vi "OBJ_LOGIN_scan_barcode.vi"(8 "error_in":errorcluster, 11 "all_config_info":T1={"main_ini_file"={"SQL Driver"="", "SQL Server"="", "SQL Database"="", "SQL UID"="", "User table"="", "Reference table"="", "default language"="", "SCANNER COM port"=0, "SCANNER Baud rate"=0, "SCANNER Data bits"=0, "SCANNER Pairity"=enum."None", "SCANNER Stop bits"=10, "SCANNER Flow control"=0, "SCANNER Termination char"=0, "MD-L COM port"=0, "MD-L Baud rate"=0, "MD-L Data bits"=0, "MD-L Pairity"=enum."None", "MD-L Stop bits"=10, "MD-L Flow control"=0, "MD-L Termination char"=0, "MD-R COM port"=0, "MD-R Baud rate"=0, "MD-R Data bits"=0, "MD-R Pairity"=enum."None", "MD-R Stop bits"=10, "MD-R Flow control"=0, "MD-R Termination char"=0, "logout timeout [ms]"=0}, "SQL Password"="", "queue_refnums"={"MAIN_queue"=refnum, "SCANNER_queue"=refnum, "SCANNER_login"=refnum, "MD_L_queue"=refnum, "MD_L_data"=refnum, "MD_R_queue"=refnum, "MD_R_data"=refnum, "OBJ_GUI_TIMER_queue"=refnum}} {"main_ini_file"."MD-R Flow control" items=["None"=0, "XON/XOFF"=1, "RTS/CTS"=2, "DTR/DSR"=4]; "main_ini_file"."MD-R Stop bits" items=["1.0"=10, "1.5"=15, "2.0"=20]; "main_ini_file"."MD-L Flow control" items=["None"=0, "XON/XOFF"=1, "RTS/CTS"=2, "DTR/DSR"=4]; "main_ini_file"."MD-L Stop bits" items=["1.0"=10, "1.5"=15, "2.0"=20]; "main_ini_file"."SCANNER Flow control" items=["None"=0, "XON/XOFF"=1, "RTS/CTS"=2, "DTR/DSR"=4]; "main_ini_file"."SCANNER Stop bits" items=["1.0"=10, "1.5"=15, "2.0"=20]}) -> (0 "error_out":errorcluster, 2 "Canceled?":bool, 3 "barcode":string)   [LabVIEW 2020]
uses:
  ini/typedef/OBJ_all_config_info.ctl
  ini/typedef/OBJ_main_ini_file.ctl
  queues/typedef/OBJ_queue_refnums.ctl
  queues/typedef/OBJ_MAIN_queue_element.ctl
  OBJ_MAIN_sequence_state.ctl
  queues/typedef/OBJ_SCANNER_queue_element.ctl
  SCANNER/OBJ_SCANNER_sequence_state.ctl
  queues/typedef/OBJ_MD_queue_element.ctl
  MEASURING_DEVICE/OBJ_MD_sequence_state.ctl
  queues/typedef/OBJ_GUI_TIMER_queue_element.ctl
  GUI_TIMER/OBJ_GUI_TIMER_sequence_state.ctl
  _misc/AULocalize/SubVIs/RegisterVI.vi
panel:
  out "waiting_for_barcode_scan_msg":string caption="(ий)Waiting for barcode scan..."
  in  "cancel_barcode_scan":bool
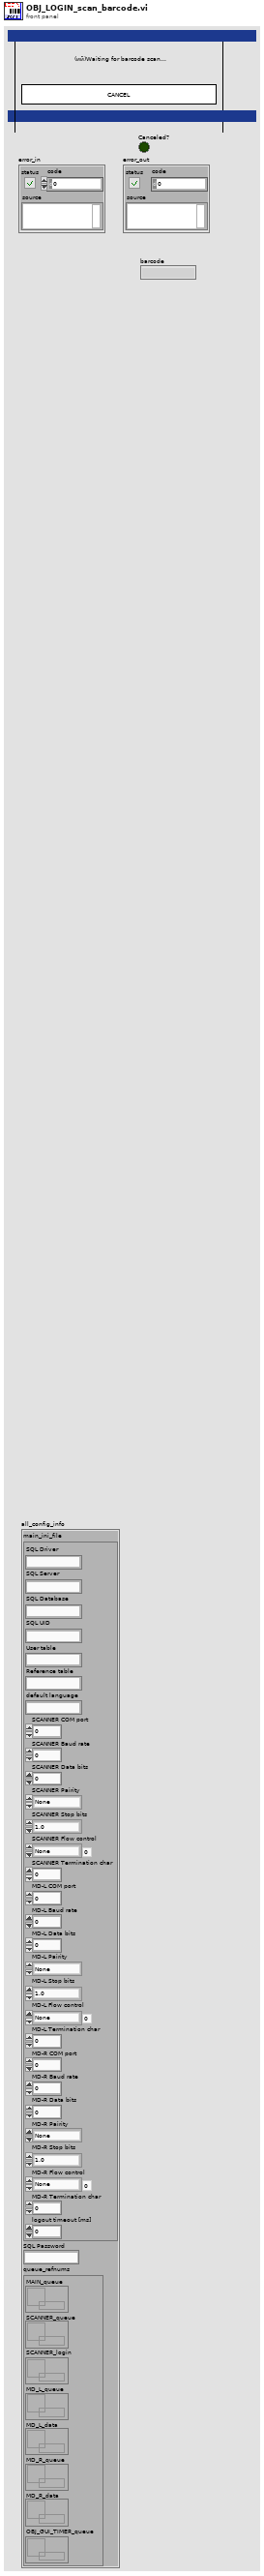
[diagram p1: front panel]
types:
  T1 = typedef "OBJ_all_config_info.ctl" = cluster{"main_ini_file":T2, "SQL Password":string, "queue_refnums":T3}
  T2 = typedef "OBJ_main_ini_file.ctl" = cluster{"SQL Driver":string, "SQL Server":string, "SQL Database":string, "SQL UID":string, "User table":string, "Reference table":string, "default language":string, "SCANNER COM port":u16, "SCANNER Baud rate":u32, "SCANNER Data bits":u16, "SCANNER Pairity":enum16{"None", "Odd", "Even", "Mark", "Space"}, "SCANNER Stop bits":u16, "SCANNER Flow control":u16, "SCANNER Termination char":u8, "MD-L COM port":u16, "MD-L Baud rate":u32, "MD-L Data bits":u16, "MD-L Pairity":enum16{"None", "Odd", "Even", "Mark", "Space"}, "MD-L Stop bits":u16, "MD-L Flow control":u16, "MD-L Termination char":u8, "MD-R COM port":u16, "MD-R Baud rate":u32, "MD-R Data bits":u16, "MD-R Pairity":enum16{"None", "Odd", "Even", "Mark", "Space"}, "MD-R Stop bits":u16, "MD-R Flow control":u16, "MD-R Termination char":u8, "logout timeout [ms]":i32}
  T3 = typedef "OBJ_queue_refnums.ctl" = cluster{"MAIN_queue":refnum<queue>, "SCANNER_queue":refnum<queue>, "SCANNER_login":refnum<queue>, "MD_L_queue":refnum<queue>, "MD_L_data":refnum<queue>, "MD_R_queue":refnum<queue>, "MD_R_data":refnum<queue>, "OBJ_GUI_TIMER_queue":refnum<queue>}
  T4 = typedef "OBJ_SCANNER_queue_element.ctl" = cluster{"state":T5, "variable":variant}
  T5 = typedef "OBJ_SCANNER_sequence_state.ctl" = enum16{"initialize", "get_next_state", "read", "error", "stop"}
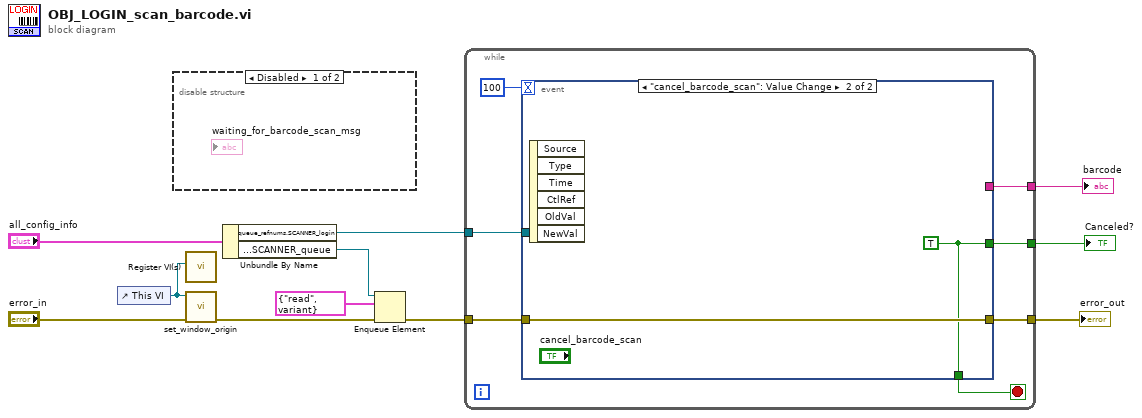
[diagram p0: block diagram]
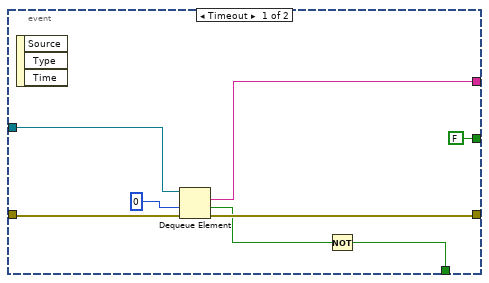
[diagram p3: hidden frame]
diagram:
  n1 = control-ref of="This VI"() -> (w1:refnum<vi>)
  n2 = disable-structure shown="Disabled" {
    frame Disabled {
    }
    frame Enabled {
    }
  }
  n3 = call-poly "Register VI(s).vi"("VI Ref"=w1) -> ()  [unwired: 9 in, 2 out]
  n4 = call "set_window_origin.vi"("error_in"="error_in", "this_vi_reference"=w1) -> ("error_out"=w6:errorcluster)  [unwired: 9 in]
  n5 = Unbundle By Name("all_config_info") -> ("queue_refnums.SCANNER_login"=w8:refnum<queue>, "queue_refnums.SCANNER_queue"=w4:refnum<queue>)
  n6 = Enqueue Element(queue=w4, element=T4 {"state"=enum."read", "variable"=variant}, error in (no error)=w6) -> (error out=w5:errorcluster)  [unwired: 1 in, 2 out]
  n7 = while {
    tunnel: w5 -> [w18]
    tunnel: [w17] -> w11
    tunnel: w8 -> [w14]
    tunnel: [w13] -> w7
    tunnel: [w12] -> w3
    stop <- w15 stop-if-true
    n8 = event shown="[1] \"cancel_barcode_scan\": Value Change" {
      selector: _ -> [_ _]
      dyn-events: _ -> [_ _]
      timeout: 100 -> [_ _]
      tunnel: w18 -> [w25 w28]
      tunnel: [w24 w28] -> w17
      tunnel: [w20 w27] -> w15
      tunnel: w14 -> [w26 _]
      tunnel: [w21 _] -> w13
      tunnel: [FALSE w27] -> w12
      event Timeout {
        n9 = event-data() -> ()  [unwired: 1 in, 3 out]
        n10 = Dequeue Element(queue=w26, timeout in ms (-1)=0, error in (no error)=w25) -> (element=w21:string, timed out?=w22:bool, error out=w24:errorcluster)  [unwired: 1 out]
        n11 = Not(x=w22) -> (.not. x?=w20:bool)
      }
      event "cancel_barcode_scan": Value Change {
        w27 = TRUE
        n12 = event-data() -> ()  [unwired: 1 in, 6 out]
      }
    }
  }
  "error_out" <- w11
  "barcode" <- w7
  "Canceled?" <- w3
